vi "rms_minus_dc.vi"   [LabVIEW 2013]
panel:
  # "3D RMS in last element"
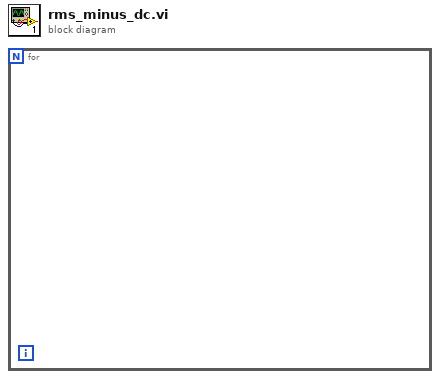
[diagram p0: block diagram]
diagram:
  n1 = for {
  }
